vi "Gserver-close.vi"(8 "error in (no error)":errorcluster, 11 "Gserver in":refnum<class "Gserver.lvclass">) -> (0 "error out":errorcluster, 3 "Gserver out":refnum<class "Gserver.lvclass">)   [LabVIEW 2020, in "Sgraph_lib_V1.lvlib" / "Gserver.lvclass"]
doc: "End the Gserver service"
uses:
  Gserver.lvclass
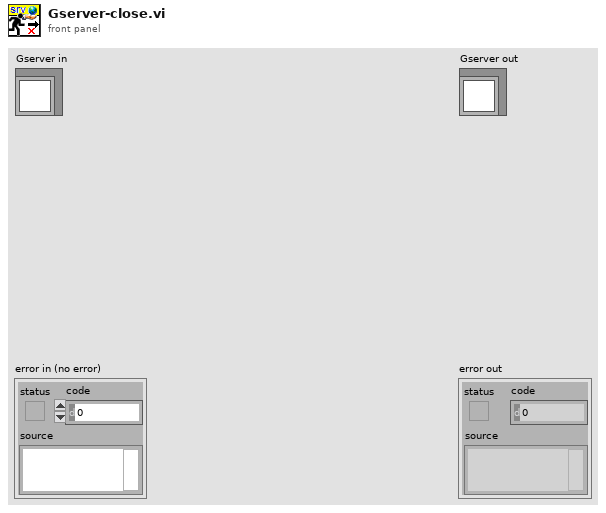
[diagram p1: front panel]
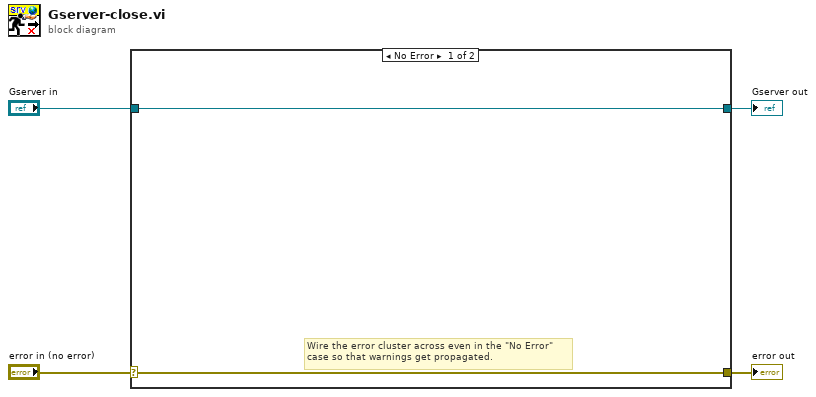
[diagram p0: block diagram]
diagram:
  n1 = case shown="No Error" "error in (no error)" {
    selector: "error in (no error)" -> [w5 w8]
    tunnel: [w5 w8] -> w3
    tunnel: [w6 w7] -> w1
    tunnel: "Gserver in" -> [w6 w7]
    frame No Error {
      # "Wire the error cluster across even in the \"No Error\"\ncase so that warnings get propagated."
    }
    frame Error {
    }
  }
  "error out" <- w3
  "Gserver out" <- w1
